vi "TDMS Data Logger.vi"(7 "File Storage Settings":T1={"Data Repository"=path "M:/data", "File Name Prefix (no spaces)"="logger", "Approximate File Size (kB)"=1000.0}, 8 "error in (no error)":errorcluster, 10 "Attributes":T2, 11 "Waveforms":waveform(sgl)[](array[waveform])) -> (0 "error out":errorcluster)   [LabVIEW 2013]
doc: "Statnett PMU Reference Library\nWrites data to TDMS file. Makes also checks if file exists and inside size limits"
panel:
  # "INPUT"
  # "INTERMEDIATE"
  # "OUTPUT"
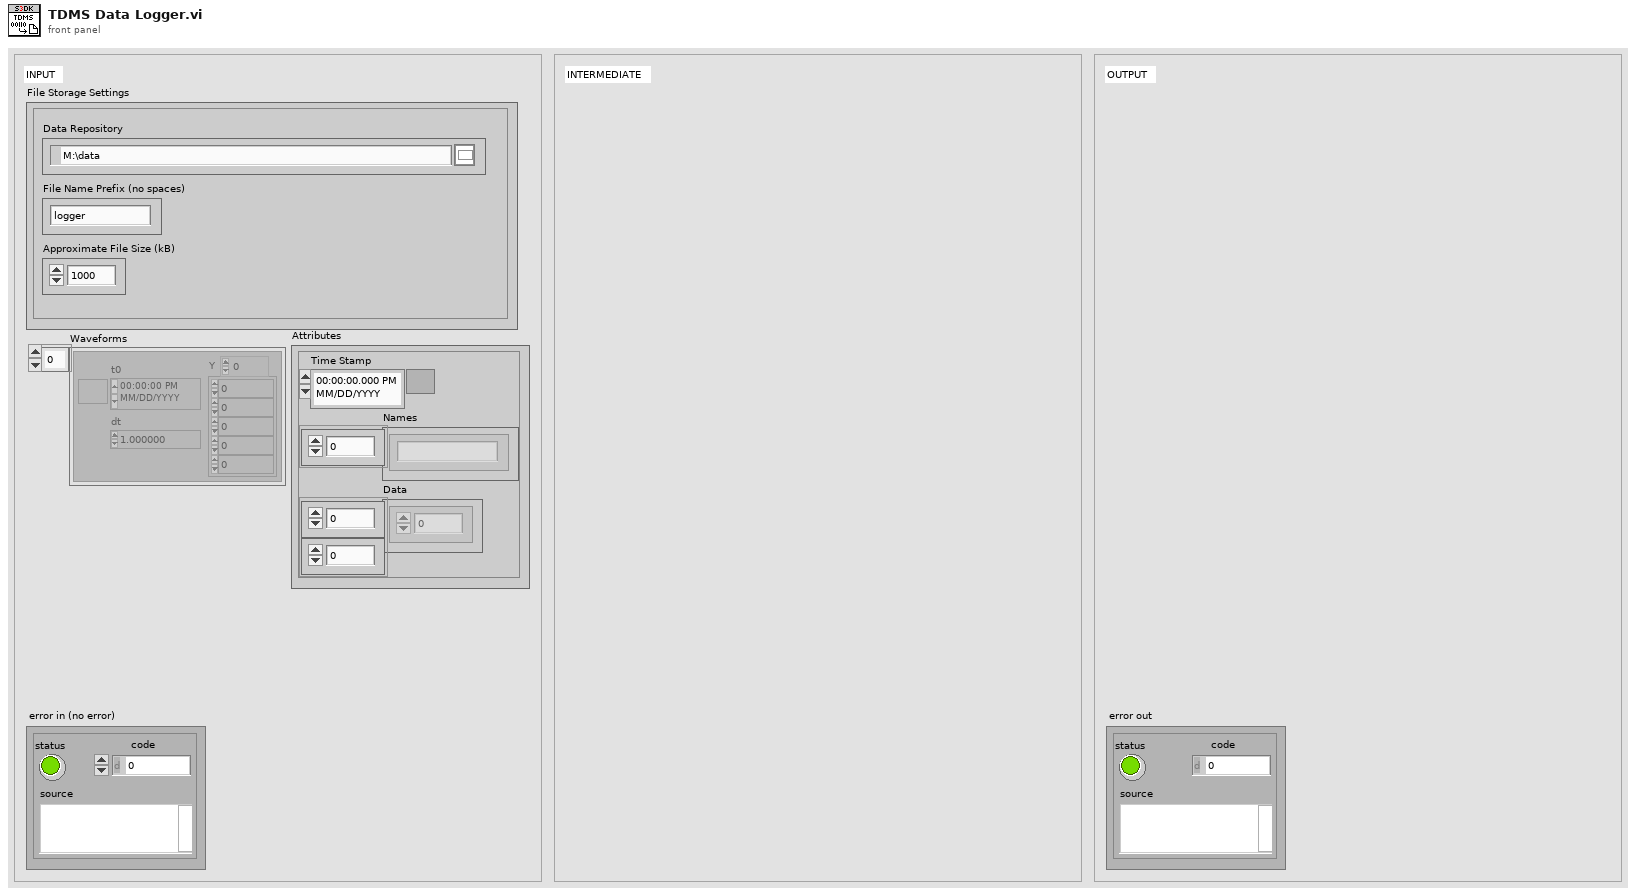
[diagram p1: front panel]
types:
  T1 = cluster{"Data Repository":path, "File Name Prefix (no spaces)":string, "Approximate File Size (kB)":dbl}
  T2 = cluster{"Time Stamp":timestamp, "Names":string[], "Data":dbl[][]}
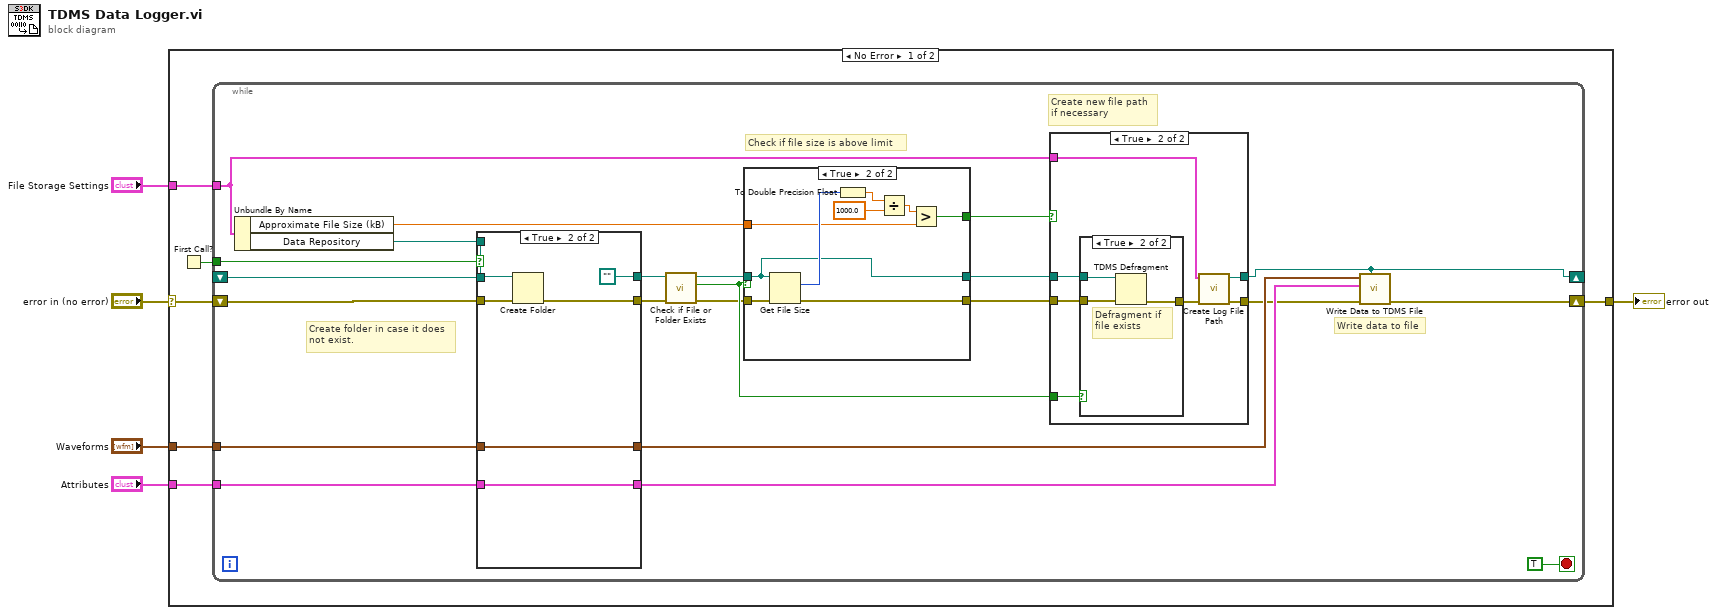
[diagram p0: block diagram]
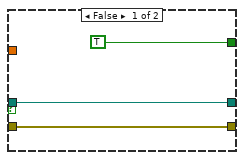
[diagram p4: hidden frame]
diagram:
  n1 = case shown="No Error" "error in (no error)" {
    selector: "error in (no error)" -> [w7 w69]
    tunnel: [w6 w69] -> w4
    tunnel: "File Storage Settings" -> [w10 _]
    tunnel: "Waveforms" -> [w9 _]
    tunnel: "Attributes" -> [w8 _]
    frame No Error {
      n2 = First Call?() -> (First Call?: T/F=w11:bool)
      n3 = while {
        tunnel: w10 -> [w27]
        shift-right: [w25] -> _
        shift-left: _ -> [w32]
        tunnel: w11 -> [w33]
        tunnel: w9 -> [w20]
        tunnel: w8 -> [w18]
        shift-right: [w13] -> w6
        shift-left: w7 -> [w17]
        stop <- TRUE stop-if-true
        # "Write data to file"
        # "Create new file path\nif necessary"
        # "Check if file size is above limit"
        # "Create folder in case it does\nnot exist."
        n4 = Unbundle By Name(w27) -> ("Approximate File Size (kB)"=w29:dbl, "Data Repository"=w22:path)
        n5 = case shown="True" w33 {
          tunnel: w32 -> [w62 _]
          tunnel: w22 -> [_ w68]
          tunnel: [w62 path ""] -> w31
          tunnel: [w61 w66] -> w21
          tunnel: w20 -> [w61 w66]
          tunnel: [w60 w65] -> w19
          tunnel: w18 -> [w60 w65]
          tunnel: w17 -> [w59 w64]
          tunnel: [w59 w63] -> w16
          frame False {
          }
          frame True {
            n6 = Create Folder(path (use dialog)=w68, error in=w64) -> (error out=w63:errorcluster)  [unwired: 1 in, 2 out]
          }
        }
        n7 = call <vilib>:"Check if File or Folder Exists.vi"("error in (no error)"=w16, "path"=w31) -> ("error out"=w15:errorcluster, "file or folder exists?"=w23:bool, "dup path"=w30:path)  [unwired: 7 in]
        n8 = case shown="True" w23 {
          tunnel: w30 -> [w48 w53]
          tunnel: w29 -> [_ w51]
          tunnel: [TRUE w54] -> w28
          tunnel: [w48 w53] -> w26
          tunnel: w15 -> [w47 w52]
          tunnel: [w47 w50] -> w14
          frame False {
          }
          frame True {
            n9 = Get File Size(file=w53, error in=w52) -> (size (in bytes)=w58:i64, 0:w50:errorcluster)  [unwired: 1 out]
            n10 = To Double Precision Float(number=w58) -> (double precision float=w57:dbl)
            n11 = Divide(x=w57, y=1000.0) -> (x/y=w55:dbl)
            n12 = Greater?(x=w55, y=w51) -> (0:w54:bool)
          }
        }
        n13 = case shown="True" w28 {
          tunnel: w27 -> [_ w42]
          tunnel: [w35 w41] -> w25
          tunnel: w26 -> [w35 w40]
          tunnel: w23 -> [_ w39]
          tunnel: w14 -> [w34 w38]
          tunnel: [w34 w36] -> w12
          frame False {
          }
          frame True {
            n14 = case shown="True" w39 {
              tunnel: w40 -> [_ w46]
              tunnel: w38 -> [w43 w45]
              tunnel: [w43 w44] -> w37
              frame False {
              }
              frame True {
                # "Defragment if \nfile exists"
                n15 = TDMS Defragment(4:w45, 7:w46) -> (0:w44:errorcluster)
              }
            }
            n16 = call "Create Log File Path.vi"("error in (no error)"=w37, "File Storage Settings"=w42) -> ("error out"=w36:errorcluster, "Path"=w41:path)  [unwired: 8 in]
          }
        }
        n17 = call "Write Data to TDMS File.vi"("TDMS File Path"=w25, "error in (no error)"=w12, "Attributes"=w19, "Waveforms"=w21) -> ("error out"=w13:errorcluster)  [unwired: 7 in]
      }
    }
    frame Error {
    }
  }
  "error out" <- w4
